vi "TrainingAlgorithm.vi"(0 "Tolerance Range (in decimal, not %)":dbl=0.15 format="%#_13g", 1 "LINX Resource":T1, 2 "Error In":errorcluster, 3 "Delay Time (s)":dbl=0.05, 4 "Target \nOutput":i32, 5 "Arduino Digital Outputs":u8[](array[numeric]), 7 "Most Erroneous\nPin Index Number":i32) -> (14 "[unwanted/total]^2":dbl, 16 "Error Out":errorcluster, 17 "LINX Resource 2":T1)   [LabVIEW 2018]
uses:
  <vilib>/MakerHub/LINX/Private/Type Defs/LINX Ref.ctl
  <vilib>/MakerHub/LINX/Private/Type Defs/Platform.ctl
  <vilib>/MakerHub/LINX/Private/Type Defs/Interface.ctl
  <vilib>/MakerHub/LINX/Private/Device/Type Defs/LINX Device Config.ctl
  <vilib>/MakerHub/LINX/Private/Device/Type Defs/TCP Config.ctl
  <vilib>/MakerHub/LINX/Private/Device/Type Defs/Channels.ctl
  <vilib>/MakerHub/LINX/Public/Peripherals/Digital/Digital Write N Chans.vi
  <vilib>/MakerHub/LINX/Private/Local IO/LinxDigitalWrite.vi
  <vilib>/MakerHub/LINX/Public/Utilities/Check Channel.vi
  <vilib>/MakerHub/LINX/Private/Utilties/Generate Error.vi
  GlobalVariables/CurrentLevelGlobal.vi
  GlobalVariables/Voltage Level Global.vi
  GlobalVariables/SetVoltagGlobal.vi
  GlobalVariables/GlobalStop.vi
  <vilib>/MakerHub/LINX/LMH-LINX.lvlib
  <vilib>/MakerHub/LINX/Private/Device/Device.lvlib
panel:
  out "Binary Inputs into\nLogic Block":bool[](array[boolean])
  out "I/V Current":dbl format="%#_13g"
  out "I/V Initial":dbl format="%#_13g"
  out "Counter":dbl format="%#_13g"
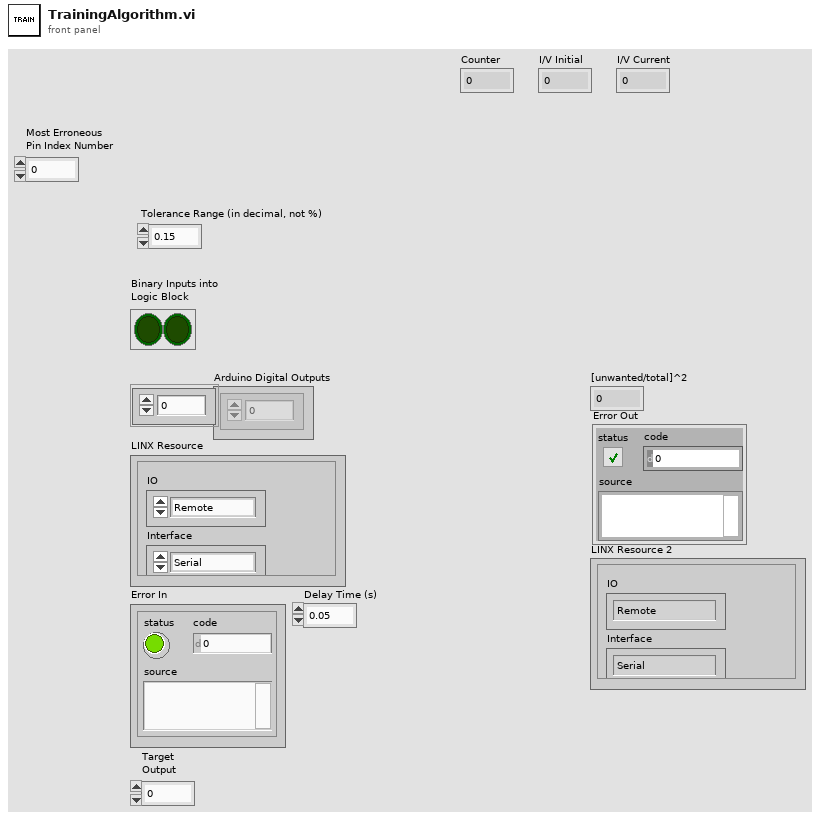
[diagram p1: front panel]
types:
  T1 = typedef "LMH-LINX.lvlib/LINX Ref.ctl" = cluster{"IO":T2, "Interface":T3, "LINX Device Config":T4}
  T2 = typedef "LMH-LINX.lvlib/Platform.ctl" = enum16{"Remote", "Local"}
  T3 = typedef "LMH-LINX.lvlib/Interface.ctl" = enum16{"Serial", "TCP"}
  T4 = typedef "LMH-LINX.lvlib/Device.lvlib/LINX Device Config.ctl" = cluster{"Interface":T3, "COM Port":refnum<visa-resource-name>, "TCP Configuration":T5, "Device Family":u8, "Device ID":u8, "Device Name":string, "TCP Ref":refnum<k5>, "Channels":T6}
  T5 = typedef "LMH-LINX.lvlib/Device.lvlib/TCP Config.ctl" = cluster{"IP Address":string, "Port":u16}
  T6 = typedef "LMH-LINX.lvlib/Channels.ctl" = cluster{"DI":u8[], "DO":u8[], "AI":u8[], "AO":u8[], "PWM":u8[], "QE":u8[], "UART":u8[], "I2C 2":u8[], "SPI":u8[], "CAN":u8[], "Servo":u8[], "AI Ref (V)":dbl, "AI Resolution (Bits)":u8, "AO Ref (V)":dbl, "AO Resolution (Bits)":u8}
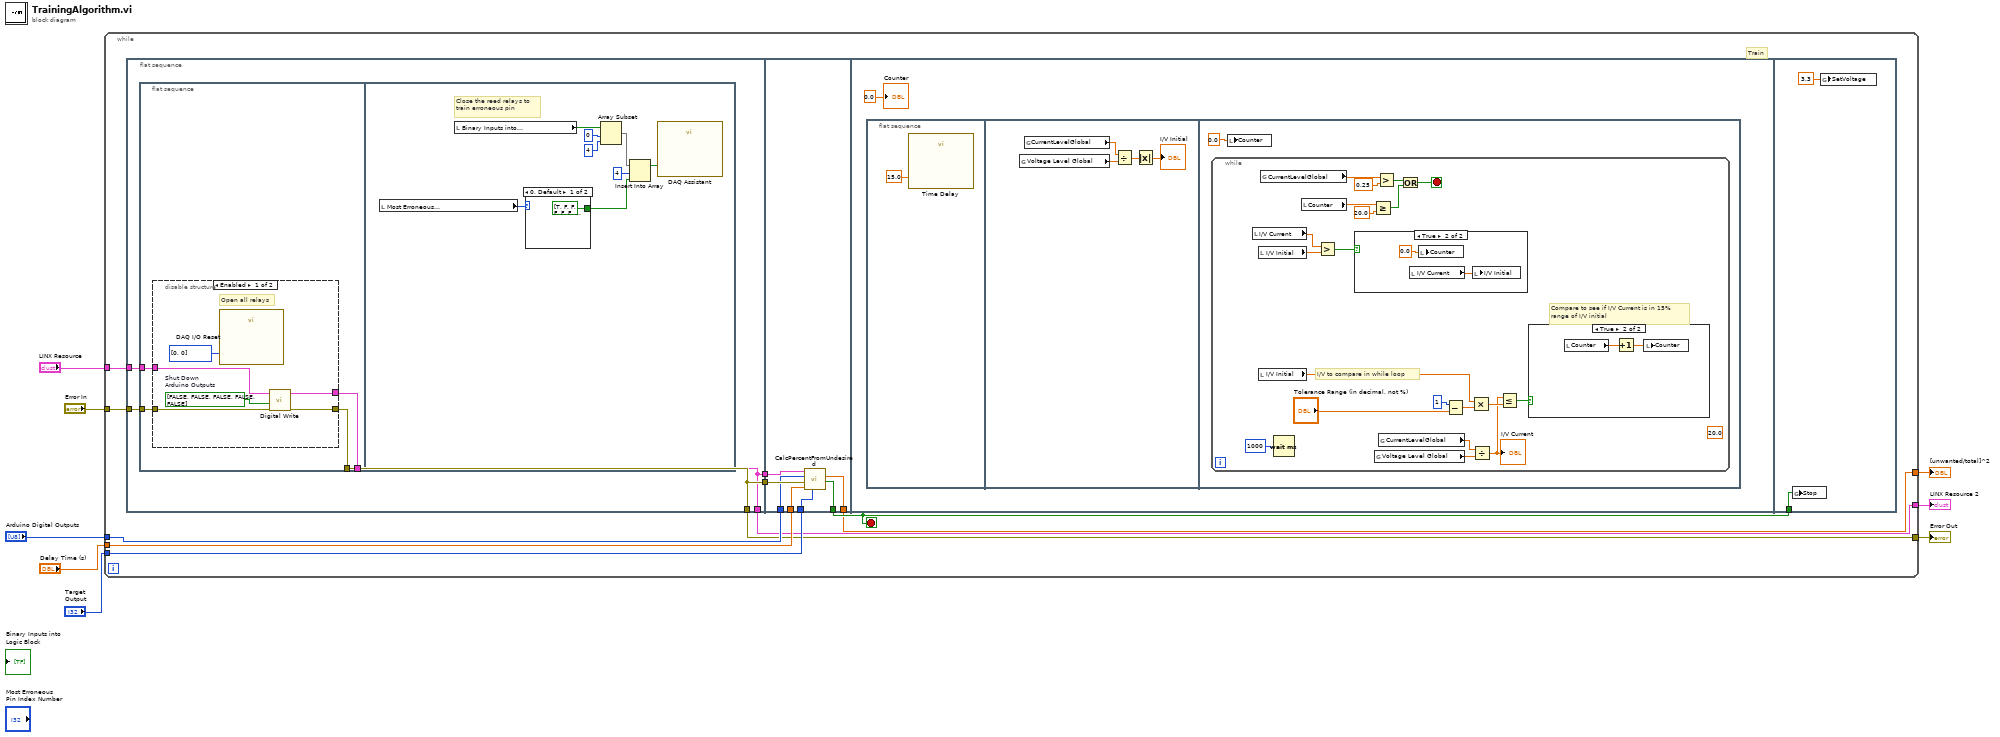
[diagram p0: block diagram]
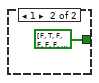
[diagram p3: hidden frame]
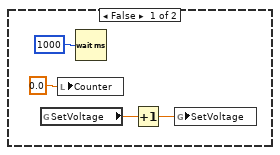
[diagram p5: hidden frame]
diagram:
  n1 = while {
    tunnel: [w18] -> w8
    tunnel: "Arduino Digital Outputs" -> [w15]
    tunnel: "LINX Resource" -> [w14]
    tunnel: "Error In" -> [w13]
    tunnel: "Delay Time (s)" -> [w12]
    tunnel: "Target \nOutput" -> [w11]
    tunnel: [w10] -> w2
    tunnel: [w9] -> w1
    stop <- w19 stop-if-true
    # "Train"
    n2 = flat-sequence {
      tunnel: [w20] -> w17
      tunnel: [w21] -> w16
      tunnel: w14 -> [w23]
      tunnel: w13 -> [w22]
      tunnel: [w21] -> w10
      tunnel: [w20] -> w9
      tunnel: [w52] -> w19
      tunnel: [w51] -> w18
      tunnel: w17 -> [w50]
      tunnel: w16 -> [w49]
      tunnel: w15 -> [w48]
      tunnel: w12 -> [w47]
      tunnel: w11 -> [w46]
      tunnel: w19 -> [w88]
      frame #0 {
        n3 = flat-sequence {
          tunnel: [w27] -> w20
          tunnel: [w26] -> w21
          tunnel: w23 -> [w25]
          tunnel: w22 -> [w24]
          frame #0 {
            n4 = disable-structure shown="Enabled" {
              disable-tunnel: [w32 w35] -> w27
              disable-tunnel: [w31 w34] -> w26
              disable-tunnel: w25 -> [w29 _]
              disable-tunnel: w24 -> [w28 _]
              frame Enabled {
                w33 = bool[] [FALSE, FALSE, FALSE, FALSE, FALSE]  # Shut Down  Arduino Outputs
                # "Open all relays"
                n5 = call "DAQ I/O Reset"("data"=u32[] [0, 0]) -> ()  [unwired: 17 in, 2 out]
                n6 = call-poly <vilib>:"Digital Write.vi"("Error In"=w28, "Values"=w33, "LINX Resource"=w29) -> ("Error Out"=w31:errorcluster, "LINX Resource"=w32:T1)  [unwired: 7 in]
              }
              frame Disabled {
              }
            }
          }
          frame #1 {
            # "Close the reed relays to\ntrain erroneous pin"
            n7 = local read "Most Erroneous\nPin Index Number"() -> (w42:i32)
            n8 = local read "Binary Inputs into\nLogic Block"() -> (w39:bool[])
            n9 = case shown="0, Default" w42 {
              tunnel: [bool[] [TRUE, FALSE, FALSE, FALSE, FALSE, FALSE, FALSE, FALSE] bool[] [FALSE, TRUE, FALSE, FALSE, FALSE, FALSE, FALSE, FALSE]] -> w40
              frame 0, Default {
              }
              frame 1 {
              }
            }
            n10 = Array Subset(array=w39, index=0, length=4) -> (w36:bool[])
            n11 = Insert Into Array(array=w36, index=4, new element=w40) -> (w41:bool[])
            n12 = call "DAQ Assistant"("data"=w41) -> ()  [unwired: 17 in, 2 out]
          }
        }
      }
      frame #1 {
        n13 = call "CalcPercentFromUndesired.vi"("Target \nOutput"=w46, "Delay Time (s)"=w47, "Error In"=w49, "Arduino Digital Outputs"=w48, "LINX Resource In"=w50) -> ("Positive values"=w52:bool, "[unwanted/total]^2"=w51:dbl)  [unwired: 5 in]
      }
      frame #2 {
        n14 = flat-sequence {
          frame #0 {
            n15 = call "Time Delay"("Delay Time (s)"=15.0) -> ()  [unwired: 10 in, 1 out]
          }
          frame #1 {
            n16 = global read "Voltage Level Global.vi" "Voltage Level Global"() -> (w55:dbl)
            n17 = global read "CurrentLevelGlobal.vi" "CurrentLevelGlobal"() -> (w56:dbl)
            n18 = Divide(x=w56, y=w55) -> (x/y=w57:dbl)
            n19 = Absolute Value(x=w57) -> (abs(x)=→"I/V Initial":dbl)
          }
          frame #2 {
            n20 = while {
              stop <- w74 stop-if-true
              (unwired) 20.0
              # "I/V to compare in while loop"
              # "Compare to see if I/V Current is in 15%\nrange of I/V initial"
              n21 = local read "I/V Current"() -> (w73:dbl)
              n22 = local read "I/V Initial"() -> (w72:dbl)
              n23 = local read "I/V Initial"() -> (w70:dbl)
              n24 = global read "CurrentLevelGlobal.vi" "CurrentLevelGlobal"() -> (w61:dbl)
              n25 = Wait (ms)(milliseconds to wait=1000) -> ()  [unwired: 1 out]
              n26 = local read "Counter"() -> (w79:dbl)
              n27 = Greater?(x=w73, y=w72) -> (0:w71:bool)
              n28 = case shown="True" w71 {
                frame False {
                }
                frame True {
                  n29 = local read "I/V Current"() -> (w81:dbl)
                  n30 = local write "Counter"(0.0) -> ()
                  n31 = local write "I/V Initial"(w81) -> ()
                }
              }
              n32 = Greater Or Equal?(x=w79, y=20.0) -> (x >= y?=w75:bool)
              n33 = global read "Voltage Level Global.vi" "Voltage Level Global"() -> (w62:dbl)
              n34 = Greater?(x=w61, y=0.25) -> (0:w76:bool)
              n35 = global read "CurrentLevelGlobal.vi" "CurrentLevelGlobal"() -> (w63:dbl)
              n36 = Or(x=w76, y=w75) -> (x .or. y?=w74:bool)
              n37 = Subtract(x=1, y="Tolerance Range (in decimal, not %)") -> (x-y=w68:dbl)
              n38 = Multiply(x=w70, y=w68) -> (x*y=w66:dbl)
              n39 = Divide(x=w63, y=w62) -> (x/y=w64:dbl)
              "I/V Current" <- w64
              n40 = Less Or Equal?(x=w64, y=w66) -> (x <= y?=w65:bool)
              n41 = case shown="True" w65 {
                frame False {
                  n42 = global read "SetVoltagGlobal.vi" "SetVoltage"() -> (w82:dbl)
                  n43 = local write "Counter"(0.0) -> ()
                  n44 = Wait (ms)(milliseconds to wait=1000) -> ()  [unwired: 1 out]
                  n45 = Increment(x=w82) -> (x+1=w84:dbl)
                  n46 = global write "SetVoltagGlobal.vi" "SetVoltage"(w84) -> ()
                }
                frame True {
                  n47 = local read "Counter"() -> (w86:dbl)
                  n48 = Increment(x=w86) -> (x+1=w87:dbl)
                  n49 = local write "Counter"(w87) -> ()
                }
              }
            }
            n50 = local write "Counter"(0.0) -> ()
          }
        }
        "Counter" <- 0.0
      }
      frame #3 {
        n51 = global write "GlobalStop.vi" "Stop"(w88) -> ()
        n52 = global write "SetVoltagGlobal.vi" "SetVoltage"(3.3) -> ()
      }
    }
  }
  "[unwanted/total]^2" <- w8
  "Error Out" <- w2
  "LINX Resource 2" <- w1
